vi "ObtainQueue.vi"(6 "ModuleID":i32, 8 "error in (no error)":errorcluster, 9 "max queue size (-1, unlimited)":i32=-1, 10 "ModuleName":string, 11 "Initial Message":string="Initialize") -> (0 "error out":errorcluster, 3 "MessageQueue":refnum<queue>)   [LabVIEW 2018, in "AcPwrPlugins.lvlib"]
doc: "This VI creates a named queue."
uses:
  AcPwrPlugins/AcPwrPlugins.lvlib
  AcPwrPlugins/Common/clMessage.ctl
panel:
  # "This obtains a queue and\nenqueues the \"Initialize\"\nMessage"
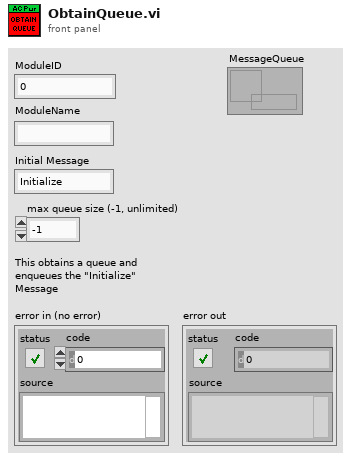
[diagram p1: front panel]
types:
  T1 = typedef "AcPwrPlugins.lvlib/clMessage.ctl" = cluster{"Message":string, "Message Data":variant}
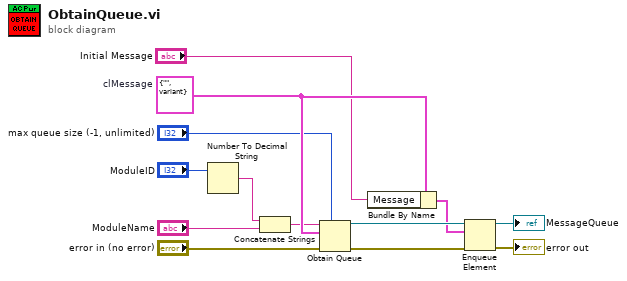
[diagram p0: block diagram]
diagram:
  w11 = T1 {"Message"="", "Message Data"=variant}  # clMessage
  n1 = Number To Decimal String(number="ModuleID") -> (decimal integer string=w4:string)  [unwired: 1 in]
  n2 = Concatenate Strings(w4, "ModuleName") -> (w2:string)
  n3 = Obtain Queue(max queue size (-1, unlimited)="max queue size (-1, unlimited)", name (unnamed)=w2, element data type=w11, error in (no error)="error in (no error)") -> (queue out=w12:refnum<queue>, error out=w8:errorcluster)  [unwired: 1 in, 1 out]
  n4 = Bundle By Name(cluster=w11, "Message"="Initial Message") -> (w9:T1)
  n5 = Enqueue Element(queue=w12, element=w9, error in (no error)=w8) -> (queue out=→"MessageQueue":refnum<queue>, error out=→"error out":errorcluster)  [unwired: 1 in, 1 out]
